vi "Write.Commit.vi"(8 "error in":errorcluster, 11 "Write in":refnum<class "Write.lvclass">) -> (0 "error out":errorcluster, 3 "Write out":refnum<class "Write.lvclass">)   [LabVIEW 2024, in "VS Plugin Data Access Engine.lvlib" / "Write.lvclass"]
uses:
  Write.lvclass
  Write.lvclass/Write.ctl
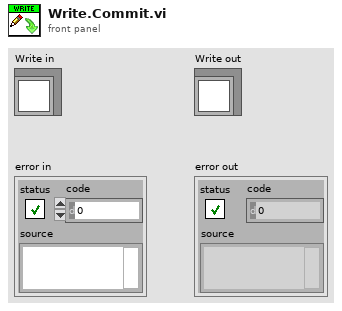
[diagram p1: front panel]
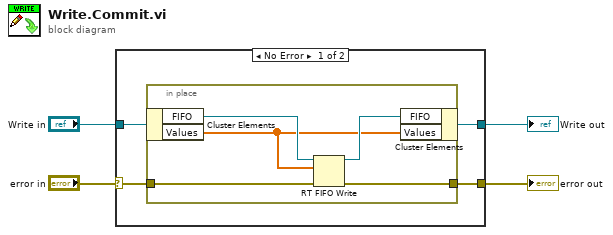
[diagram p0: block diagram]
diagram:
  n1 = case shown="No Error" "error in" {
    selector: "error in" -> [w8 w15]
    tunnel: [w7 w15] -> w3
    tunnel: [w5 w14] -> w1
    tunnel: "Write in" -> [w6 w14]
    frame No Error {
      n2 = in-place {
        in-place-border: w8 -> [w13]
        in-place-border: [w12] -> w7
        n3 = in-place-cluster #1(w6) -> ("FIFO"=w11:refnum<k33>, "Values"=w9:dbl[])
        n4 = RT FIFO Write(0:w11, 1:w9, 3:w13) -> (8:w10:refnum<k33>, 11:w12:errorcluster)  [unwired: 2 in, 2 out]
        n5 = in-place-cluster #1("FIFO"=w10, "Values"=w9) -> (w5:refnum<class "Write.lvclass">)
      }
    }
    frame Error {
    }
  }
  "error out" <- w3
  "Write out" <- w1
